vi "Manage RunTime Checkbox.vi"(6 "Change(T)/set(F)":bool, 8 "error in (no error)":errorcluster, 9 "Message Data":variant, 10 "String":string, 11 "Menu Checkbox":bool) -> (0 "error out":errorcluster, 3 "New Checkbox Value":bool)   [LabVIEW 2024, in "User Interface.lvlib"]
uses:
  User Interface.lvlib
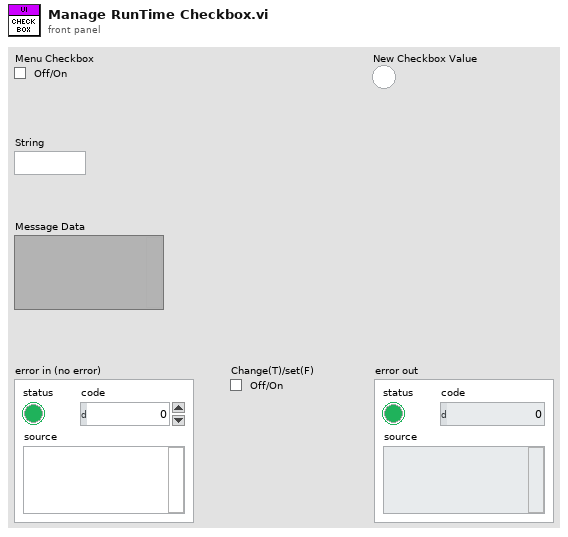
[diagram p1: front panel]
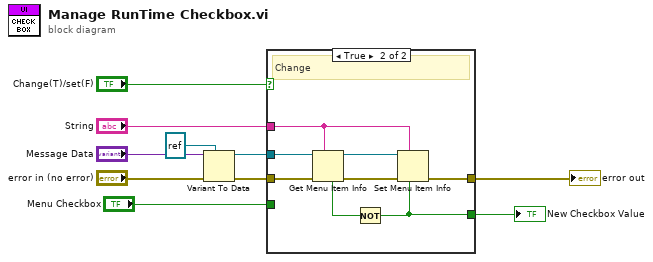
[diagram p0: block diagram]
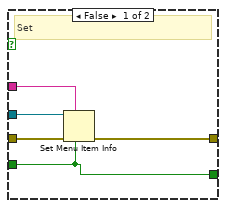
[diagram p2: hidden frame]
diagram:
  n1 = Variant To Data(error in="error in (no error)", type=refnum<k9> refnum ("MenuRef"), Variant="Message Data") -> (data=w6:refnum<k9>, error out=w4:errorcluster)
  n2 = case shown="True" "Change(T)/set(F)" {
    tunnel: "String" -> [w13 w23]
    tunnel: [w12 w22] -> w8
    tunnel: w6 -> [w14 w21]
    tunnel: w4 -> [w15 w20]
    tunnel: "Menu Checkbox" -> [w11 _]
    tunnel: [w11 w16] -> w1
    frame False {
      # "Set"
      n3 = Set Menu Item Info(6:w11, 7:w13, 8:w15, 11:w14) -> (0:w12:errorcluster)  [unwired: 3 in, 1 out]
    }
    frame True {
      # "Change"
      n4 = Get Menu Item Info(7:w23, 8:w20, 11:w21) -> (0:w18:errorcluster, 3:w19:refnum<k9>, 4:w17:bool)  [unwired: 4 out]
      n5 = Not(x=w17) -> (.not. x?=w16:bool)
      n6 = Set Menu Item Info(6:w16, 7:w23, 8:w18, 11:w19) -> (0:w22:errorcluster)  [unwired: 3 in, 1 out]
    }
  }
  "error out" <- w8
  "New Checkbox Value" <- w1
